vi "8.4.1.vi"   [LabVIEW 2018]
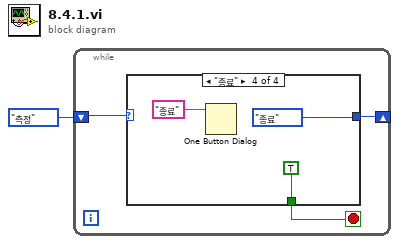
[diagram p0: block diagram]
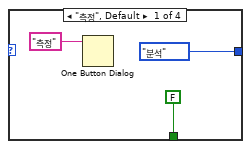
[diagram p2: hidden frame]
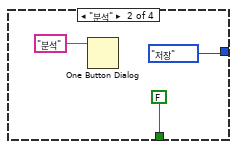
[diagram p3: hidden frame]
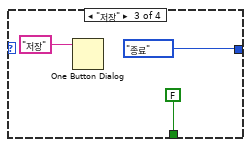
[diagram p4: hidden frame]
diagram:
  n1 = while {
    shift-right: [w3] -> _
    shift-left: enum16{"측정", "분석", "저장", "종료"}."측정" -> [w4]
    stop <- w2 stop-if-true
    n2 = case shown="\"종료\"" w4 {
      tunnel: [enum16{"측정", "분석", "저장", "종료"}."분석" enum16{"측정", "분석", "저장", "종료"}."저장" enum16{"측정", "분석", "저장", "종료"}."종료" enum16{"측정", "분석", "저장", "종료"}."종료"] -> w3
      tunnel: [FALSE FALSE FALSE TRUE] -> w2
      frame "측정", Default {
        n3 = One Button Dialog(message="측정") -> ()  [unwired: 1 in, 1 out]
      }
      frame "분석" {
        n4 = One Button Dialog(message="분석") -> ()  [unwired: 1 in, 1 out]
      }
      frame "저장" {
        n5 = One Button Dialog(message="저장") -> ()  [unwired: 1 in, 1 out]
      }
      frame "종료" {
        n6 = One Button Dialog(message="종료") -> ()  [unwired: 1 in, 1 out]
      }
    }
  }
